vi "Get Column.vi"(0 "2D Array Input":string[][](array[string]), 11 "Column Number":i32) -> (8 "1D Column Array":string[](array[string]))   [LabVIEW 2012]
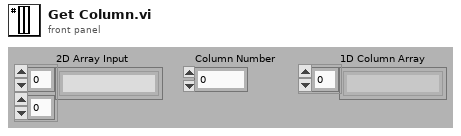
[diagram p1: front panel]
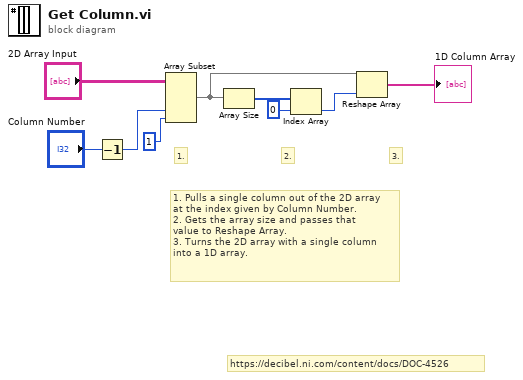
[diagram p0: block diagram]
diagram:
  # "https://decibel.ni.com/content/docs/DOC-4526"
  # "1. Pulls a single column out of the 2D array\nat the index given by Column Number. \n2. Gets the array size and passes that\nvalue to Reshape Array. \n3. Turns the 2D array with a single column \ninto a 1D array."
  # "3."
  # "2."
  # "1."
  n1 = Decrement(x="Column Number") -> (x-1=w1:i32)
  n2 = Array Subset "Array Subset"(array="2D Array Input", index (col)=w1, length (col)=1 ("length")) -> (w5:string[][])  [unwired: 2 in]
  n3 = Array Size(array=w5) -> (size(s)=w6:i32[])
  n4 = Index Array "Index Array"(array=w6, index=0) -> (element=w8:i32)
  n5 = Reshape Array "Reshape Array"(w5, w8) -> (→"1D Column Array":string[])
